vi "Patch data preview-Generate positions array.vi"(8 "Error in":errorcluster, 9 "Rows/Columns":T2={"Number of rows to generate"=6, "Number of columns to generate"=0}, 11 "Experiment Parameters":T3={"Total Number of Miniscans"=1012, "Number of Trials"=20, "Number of cycles in a trial"=344, "Number of miniscans in a frame (Y)"=44, "Number of Pixels in Miniscan (X)"=85, "Number of Frames in Each Trial"=7912, "Number of Frames in a Cycle"=23, "DwellTime (us)"=0.05, "Acquisition length (sec)"=10.0, "Variable Length"=FALSE, "Pixels in miniscan (X)"=[], "Number of lines in frame (Y)"=[]}) -> (0 "error out":errorcluster, 2 "Frames info":T1)   [LabVIEW 2020]
uses:
  User Interface/Visualisation/Patch-Vol video generator/Typedefs/Experiment Parameters.ctl
  <vilib>/Utility/miscctls.llb/LVPointTypeDef.ctl
  <userlib>/_OpenG.lib/array/array.llb/Sort 1D Array (I32)__ogtk.vi
  <userlib>/_OpenG.lib/array/array.llb/Remove Duplicates from 1D Array (I32)__ogtk.vi
  <userlib>/_OpenG.lib/array/array.llb/Delete Elements from 1D Array (I32)__ogtk.vi
panel:
  in  "Layout":i32[][](array[numeric])=[[1, 2, 2, 13], [23, 1, 9, 2], [4, 19, 21, 10], [11, 12, 20, 17], [18, 22, 7, 6], [5, 8, 15, 15]] min=1 max=100 step=1 format="Image %d"
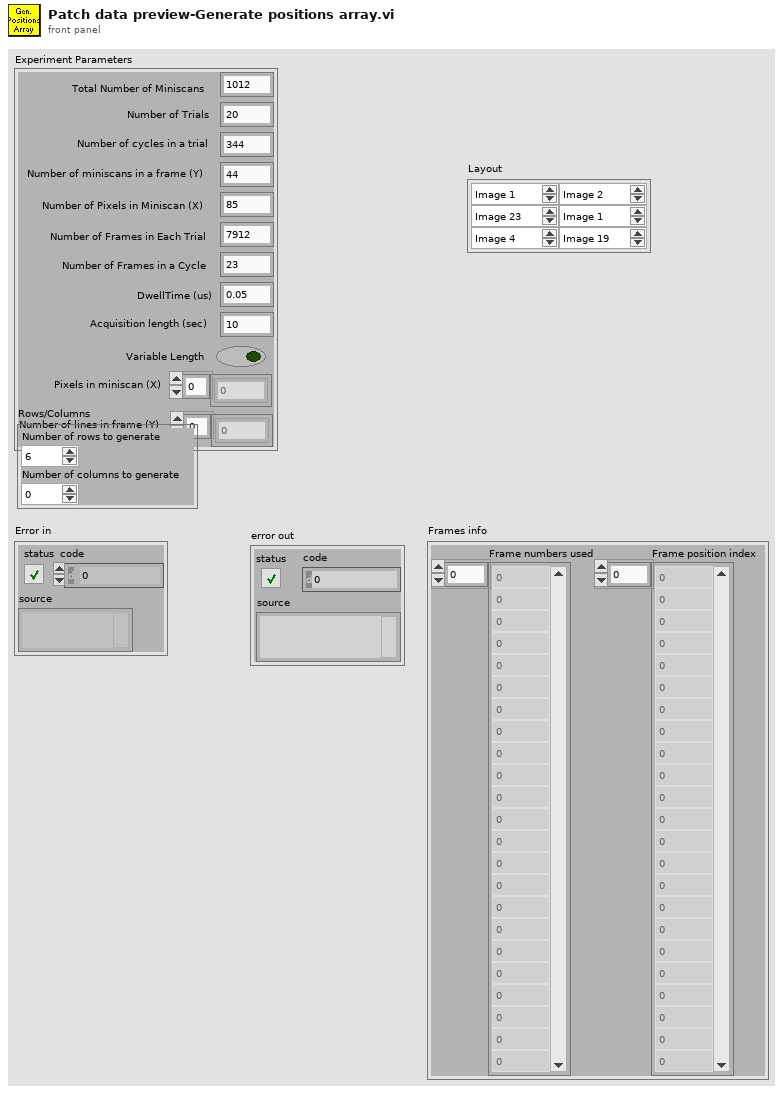
[diagram p1: front panel]
types:
  T1 = cluster{"Frame numbers used":i32[], "Frame position index":i32[]}
  T2 = cluster{"Number of rows to generate":i32, "Number of columns to generate":i32}
  T3 = typedef "Experiment Parameters.ctl" = cluster{"Total Number of Miniscans":i32, "Number of Trials":i32, "Number of cycles in a trial":i32, "Number of miniscans in a frame (Y)":i32, "Number of Pixels in Miniscan (X)":i32, "Number of Frames in Each Trial":i32, "Number of Frames in a Cycle":i32, "DwellTime (us)":dbl, "Acquisition length (sec)":dbl, "Variable Length":bool, "Pixels in miniscan (X)":dbl[], "Number of lines in frame (Y)":dbl[]}
  T4 = typedef "LVPointTypeDef.ctl" = cluster{"Horizontal":i16, "Vertical":i16}
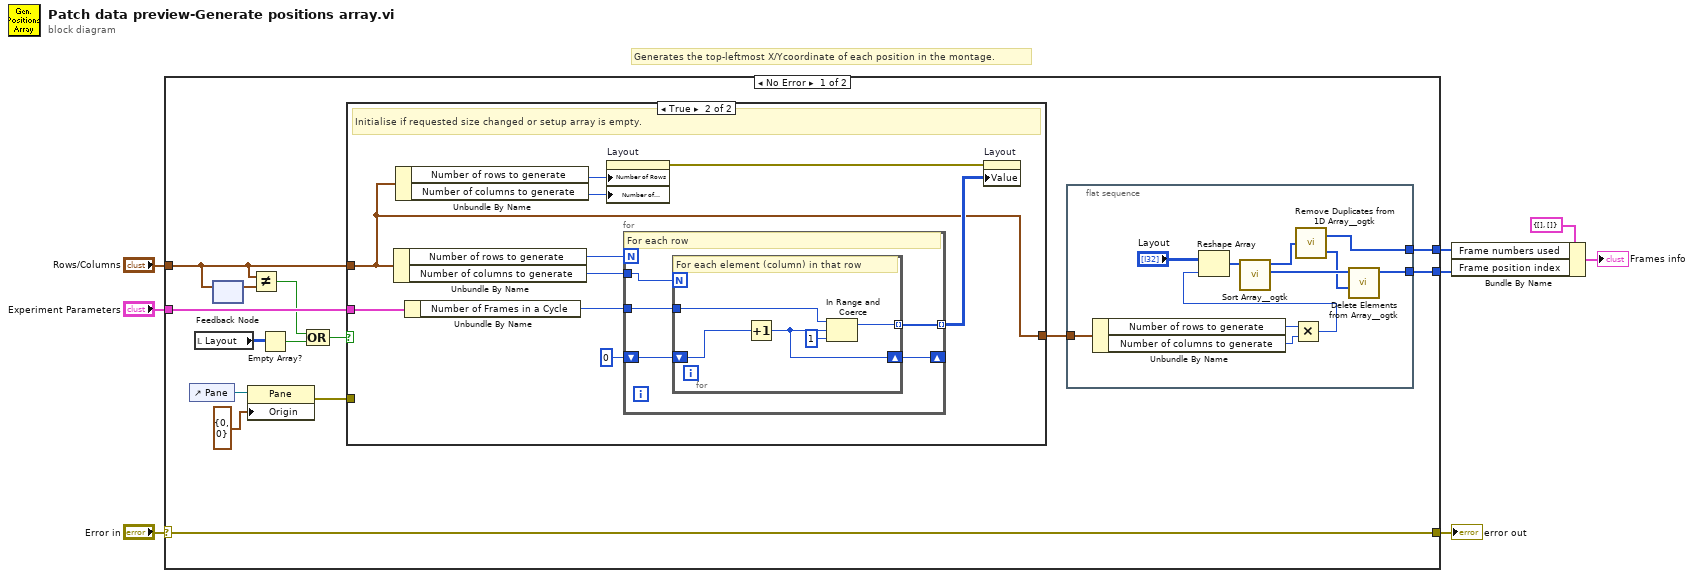
[diagram p0: block diagram]
diagram:
  # "Generates the top-leftmost X/Ycoordinate of each position in the montage."
  n1 = case shown="No Error" "Error in" {
    selector: "Error in" -> [w22 w55]
    tunnel: "Experiment Parameters" -> [w21 _]
    tunnel: [w22 w55] -> w6
    tunnel: "Rows/Columns" -> [w15 _]
    tunnel: [w20 _] -> w2
    tunnel: [w19 _] -> w3
    frame No Error {
      n2 = control-ref of="Pane"() -> (w11:refnum<vi>)
      n3 = local read "Layout"() -> (w18:i32[][])
      n4 = feedback-in #1(w15) -> ()
      n5 = feedback #1() -> (w16:T2)  [unwired: 1 in]
      n6 = property class="Pane"(reference=w11, "Origin"=T4 {"Horizontal"=0, "Vertical"=0}) -> (error out=w10:errorcluster)  [unwired: 1 in, 1 out]
      n7 = Not Equal?(x=w15, y=w16) -> (x != y?=w14:bool)
      n8 = Empty Array?(array=w18) -> (empty?=w17:bool)
      n9 = Compound Arithmetic op=OR(w14, w17) -> (w13:bool)
      n10 = case shown="True" w13 {
        tunnel: w21 -> [_ w44]
        tunnel: w15 -> [w34 w35]
        tunnel: [w34 w35] -> w12
        tunnel: w10 -> [_ _]
        frame False {
          # "Do not initialise."
        }
        frame True {
          # "Initialise if requested size changed or setup array is empty."
          n11 = Unbundle By Name(w35) -> ("Number of rows to generate"=w43:i32, "Number of columns to generate"=w42:i32)
          n12 = Unbundle By Name(w35) -> ("Number of rows to generate"=w41:i32, "Number of columns to generate"=w40:i32)
          n13 = Unbundle By Name(w44) -> ("Number of Frames in a Cycle"=w38:i32)
          n14 = property on="Layout" class="Arr (strict)"("Number of Rows"=w41, "Number of Columns"=w40) -> (error out=w39:errorcluster)  [unwired: 2 in, 1 out]
          n15 = for {
            N: w43 -> [_]
            tunnel: w42 -> [w49]
            tunnel: w38 -> [w47]
            tunnel: [w48] -> w37 mode=indexing
            shift-right: [w46] -> _
            shift-left: 0 ("lower limit") -> [w45]
            # "For each row"
            n16 = for {
              N: w49 -> [_]
              tunnel: [w53] -> w48 mode=indexing
              tunnel: w47 -> [w54]
              shift-right: [w51] -> w46
              shift-left: w45 -> [w50]
              # "For each element (column) in that row"
              n17 = Increment(x=w50) -> (x+1=w51:i32)
              n18 = In Range and Coerce(upper limit=w54, x=w51, lower limit=1) -> (coerced(x)=w53:i32)  [unwired: 1 out]
            }
          }
          n19 = property on="Layout" class="Arr (strict)"(error in=w39, "Value"=w37) -> ()  [unwired: 1 in, 2 out]
        }
      }
      n20 = flat-sequence {
        tunnel: [w33] -> w20
        tunnel: [w32] -> w19
        tunnel: w12 -> [w31]
        frame #0 {
          n21 = Unbundle By Name(w31) -> ("Number of rows to generate"=w28:i32, "Number of columns to generate"=w27:i32)
          n22 = Multiply(x=w28, y=w27) -> (x*y=w29:i32)
          n23 = Reshape Array("Layout", w29) -> (w26:i32[])
          n24 = call-poly <userlib>:"Sort Array__ogtk.vi"("Array in"=w26) -> ("Sorted Pointers"=w24:i32[], "Sorted Array out"=w25:i32[])  [unwired: 9 in]
          n25 = call-poly <userlib>:"Remove Duplicates from 1D Array__ogtk.vi"("Input Array"=w25) -> ("Output Array"=w32:i32[], "indices of removed elements"=w23:i32[])
          n26 = call-poly <userlib>:"Delete Elements from Array__ogtk.vi"("indices"=w23, "array"=w24) -> ("array w/ subset deleted"=w33:i32[])  [unwired: 8 in, 1 out]
        }
      }
    }
    frame Error {
    }
  }
  "error out" <- w6
  n27 = Bundle By Name(cluster=T1 {"Frame numbers used"=[], "Frame position index"=[]} ("Frames info"), "Frame numbers used"=w3, "Frame position index"=w2) -> (→"Frames info":T1)
